vi "set_MessageAndLabels.vi"(0 "HB_Dialog in":refnum<class "HB_Dialog.lvclass">, 5 "Message":string, 7 "T button name (\"OK\")":string="OK", 9 "F button name (\"Cancel\")":string="Cancel", 11 "error in (no error)":errorcluster) -> (4 "HB_Dialog out":refnum<class "HB_Dialog.lvclass">, 15 "error out":errorcluster)   [LabVIEW 2009, in "HB_HGF_Test.lvlib" / "HB_Dialog.lvclass"]
doc: "Set default message and button label text."
uses:
  HB_Dialog.lvclass
  HB_Dialog.lvclass/HB_Dialog.ctl
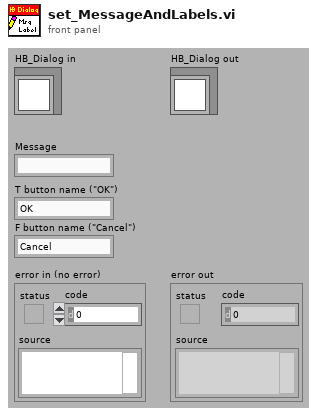
[diagram p1: front panel]
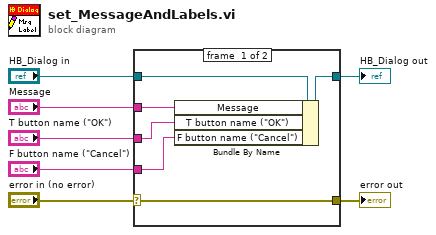
[diagram p0: block diagram]
diagram:
  n1 = case shown="No Error" "error in (no error)" {
    selector: "error in (no error)" -> [w13 w14]
    tunnel: [w13 w14] -> w6
    tunnel: [w11 w15] -> w4
    tunnel: "HB_Dialog in" -> [w12 w15]
    tunnel: "Message" -> [w10 _]
    tunnel: "T button name (\"OK\")" -> [w9 _]
    tunnel: "F button name (\"Cancel\")" -> [w8 _]
    frame #0 {
      n2 = Bundle By Name(cluster=w12, "Message"=w10, "T button name (\"OK\")"=w9, "F button name (\"Cancel\")"=w8) -> (w11:refnum<class "HB_Dialog.lvclass">)
    }
    frame #1 {
    }
  }
  "error out" <- w6
  "HB_Dialog out" <- w4
